vi "SysInfo-Get Path To App Version.vi"(0 "Path root":string, 11 "error in":errorcluster) -> (4 "Path with version":string, 8 "Path without version":path, 15 "error out":errorcluster)   [LabVIEW 2020]
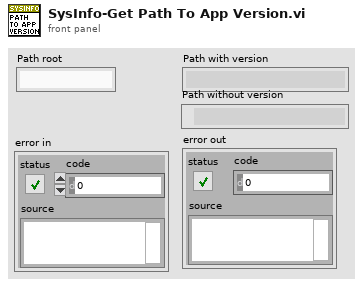
[diagram p1: front panel]
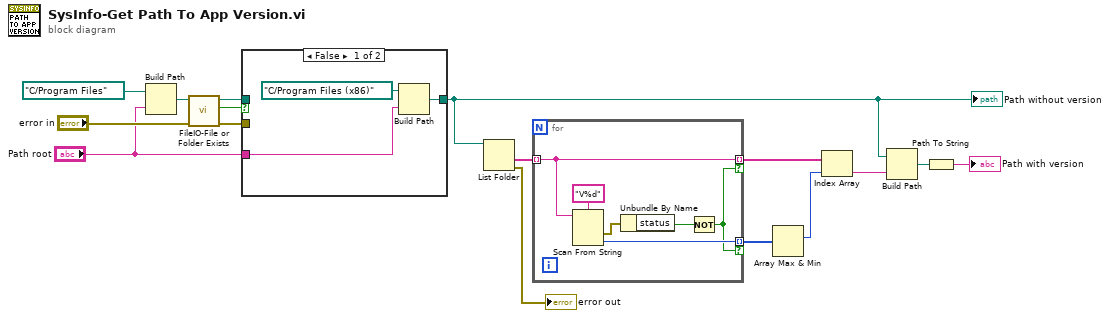
[diagram p0: block diagram]
diagram:
  n1 = Build Path(base path=path "C:/Program Files", name or relative path="Path root") -> (appended path=w7:path)
  n2 = call "FileIO-File or Folder Exists.vi"("error in (no error)"="error in", "path"=w7) -> ("error out"=w5:errorcluster, "Directory?"=w4:bool, "dup path"=w3:path)  [unwired: 6 in, 1 out]
  n3 = case shown="False" w4 {
    tunnel: w5 -> [_ _]
    tunnel: w3 -> [_ w20]
    tunnel: [w17 w20] -> w2
    tunnel: "Path root" -> [w18 _]
    frame False {
      n4 = Build Path(base path=path "C:/Program Files (x86)", name or relative path=w18) -> (appended path=w17:path)
    }
    frame True {
    }
  }
  "Path without version" <- w2
  n5 = List Folder(path=w2) -> (folder names=w16:string[], error out=→"error out":errorcluster)  [unwired: 3 in, 2 out]
  n6 = for {
    tunnel: w16 -> [w22] mode=indexing
    tunnel: [w25] -> w15 mode=indexing if=w21
    tunnel: [w22] -> w13 mode=indexing if=w21
    n7 = Scan From String(format string="V%d", input string=w22) -> (error out=w24:errorcluster, output 1=w25:i32)  [unwired: 3 in, 2 out]
    n8 = Unbundle By Name(w24) -> ("status"=w23:bool)
    n9 = Not(x=w23) -> (.not. x?=w21:bool)
  }
  n10 = Array Max & Min(array=w15) -> (max index (indices)=w14:i32)  [unwired: 3 out]
  n11 = Index Array(array=w13, index=w14) -> (element=w12:string)
  n12 = Build Path(base path=w2, name or relative path=w12) -> (appended path=w10:path)
  n13 = Path To String(path=w10) -> (string=→"Path with version":string)
